vi "ShutdownDialog.vi"() -> ()   [LabVIEW 2015]
panel:
  in  "Tab Control":enum32{"Startup", "Shutdown"}(tab)
  in  "OK Button 3":bool
  in  "Cancel Button":bool
  in  "OK Button 2":bool
  in  "OK Button":bool
  # "Startup instructions\n - ...."
  # "Shutdown instructions\n - ...."
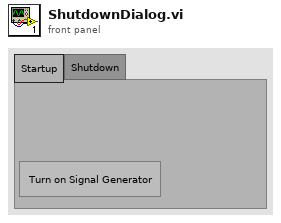
[diagram p1: front panel]
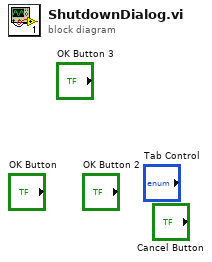
[diagram p0: block diagram]
diagram:
